vi "LLLL.vi"() -> ()   [LabVIEW 2016]
panel:
  out "Waveform Chart":u32(graph)
  in  "Knob":dbl(knob) scale=0.0..255.0
  in  "Stop Button":bool
  out "Error Out":errorcluster
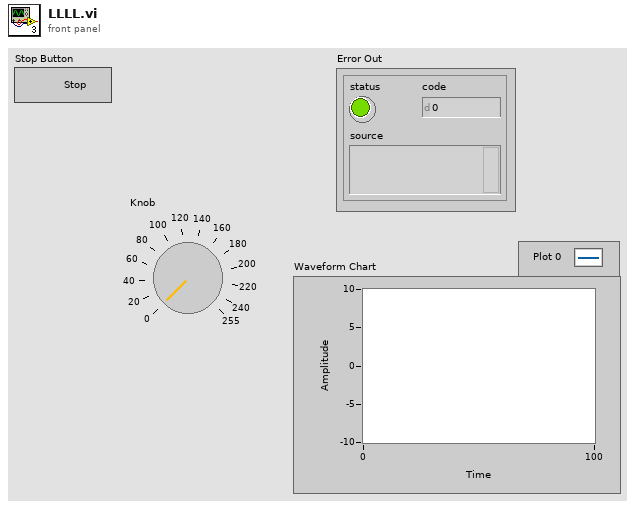
[diagram p1: front panel]
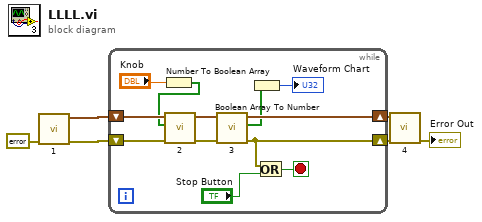
[diagram p0: block diagram]
diagram:
  n1 = call "1.vi"("Error In"=errorcluster {"status"=FALSE, "code"=0, "source"=""}) -> ("Error Out"=w6:errorcluster, "buffer"=w5:cluster{"PIPE in":i32, "PIPE OUT":i32})  [unwired: 9 in]
  n2 = while {
    shift-right: [w11] -> w3
    shift-left: w6 -> [w18]
    shift-right: [w15] -> w4
    shift-left: w5 -> [w17]
    stop <- w12 stop-if-true
    n3 = Number To Boolean Array(number="Knob") -> (Boolean array=w7:bool[])
    n4 = call <userlib>:"2.vi"("Error In"=w18, "Array"=w7, "buffer in"=w17) -> ("Error Out"=w14:errorcluster, "buffer out"=w16:cluster{"PIPE IN":i32, "PIPE OUT":i32})  [unwired: 7 in]
    n5 = call <userlib>:"3.vi"("Error In"=w14, "buffer in"=w16) -> ("Error Out"=w11:errorcluster, "lectura"=w9:bool[], "buffer out"=w15:cluster{"Pipe in":i32, "Pipe out":i32})  [unwired: 7 in]
    n6 = Boolean Array To Number(Boolean array=w9) -> (number=→"Waveform Chart":u32)
    n7 = Or(x=w11, y="Stop Button") -> (x .or. y?=w12:bool)
  }
  n8 = call <userlib>:"4.vi"("Error In"=w3, "buffer in"=w4) -> ("Error Out"=→"Error Out":errorcluster)  [unwired: 8 in, 1 out]
